vi "Insight_RW_Sweep_Start_Delay.vi"(7 "Parameter Type":enum16{"Value", "MAXimum", "MINimum", "DEFault"}(ring), 8 "error in (no error)":errorcluster, 9 "Mode (Read / Write)":enum8{"Write", "Read"}(ring), 10 "Sweep Start Delay (nsec)":dbl format="%.3g", 11 "telnet connection":T1) -> (0 "error out":errorcluster, 1 "response data":string, 2 "Sweep Start Delay (nsec)":dbl format="%.3g", 3 "telnet  connection out":T1)   [LabVIEW 2015]
doc: "Insight Photonic Solutions\n\nThis VI reads and writes the delay (nsec) of the sweep start signal to the user. Use this to synchronize data acquisition and the laser sweep.\n\nINPUTS\n\nMode - Tells the VI whether the command is a Read or a Write. (Default = Read).\nParameter Type - Tells the VI whether the command should use a Value or a keyword MAXimum, MINimum or DEFault to set the parameter value. (Default = Value).\nSweep Start Delay (nsec) - The numeric value to set the delay time between the Start Sweep Trigger and the begiining of the sweep. (Default = 0.0).\nerror in - The standard LabView Error cluster. Use this to enforce sequentiality and error tracking.\n\nOUTPUTS\n\nresponse data - the complete response string from the laser\nSweep Start Delay (nsec) - the sweep start delay written to or read from the laser\nerror out - the standard error cluster. Reports errors in reading or writing to the laser, or passes through errors from before this VI.\n\nver 1.0 - original release\nver 1.1 - return full response string and capture error if a parameter or the command is not recognized.\nver 3.2 - updated parser to accept responses from Atlas 3.1 and earlier or Atlas 3.2 and later.\nver 3.4 - accepts key word values Max, Min or Default in addition to numeric values of the parameter"
uses:
  Telnet Session.ctl
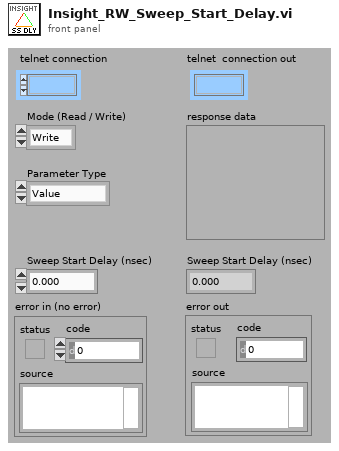
[diagram p1: front panel]
types:
  T1 = typedef "Telnet Session.ctl" = refnum<k1>
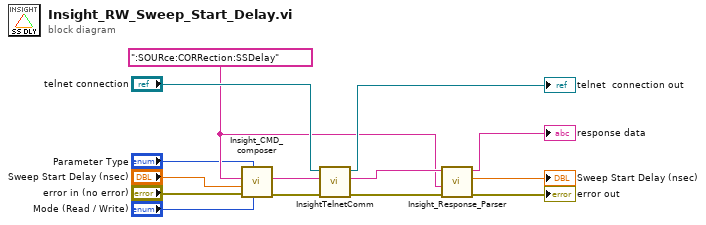
[diagram p0: block diagram]
diagram:
  w5 = ":SOURce:CORRection:SSDelay" ("String")
  n1 = call "Insight_CMD_composer.vi"("Mode (Read / Write)"="Mode (Read / Write)", "Parameter Type"="Parameter Type", "error in (no error)"="error in (no error)", "Value"="Sweep Start Delay (nsec)", "CMD"=w5) -> ("error out"=w7:errorcluster, "Command String"=w4:string)  [unwired: 5 in]
  n2 = call "InsightTelnetComm.vi"("error in"=w7, "write buffer (\"\")"=w4, "telnet connection"="telnet connection") -> ("error out"=w12:errorcluster, "response data"=w10:string, "telnet  connection out"=→"telnet  connection out":T1)  [unwired: 4 in]
  n3 = call "Insight_Response_Parser.vi"("error in (no error)"=w12, "Command String"=w5, "Laser Response In"=w10) -> ("error out"=→"error out":errorcluster, "Value"=→"Sweep Start Delay (nsec)":dbl, "Laser Response Out"=→"response data":string)  [unwired: 6 in]
